vi "ReportEnd_A131258.vi"(6 "文件重命名":bool, 8 "error in (no error)":errorcluster caption="错误输入（无错误）", 10 "文件名称":string, 11 "report in":refnum<class "NI_report.lvclass"> caption="报表输入") -> (0 "error out":errorcluster caption="错误输出")   [LabVIEW 2020]
uses:
  <vilib>/Utility/NIReport.llb/NI_report.lvclass
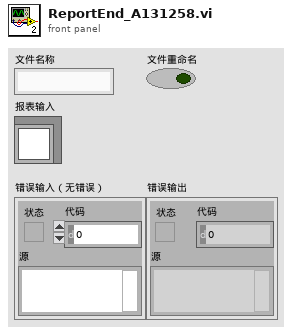
[diagram p1: front panel]
types:
  T1 = cluster{"Italic":enum16{"Italic Unchanged", "Italic On", "Italic Off"}, "Strike Through":enum16{"Strike Through Unchanged", "Strike Through On", "Strike Through Off"}, "Underline":enum16{"Underline Unchanged", "Underline On", "Underline Off"}, "Bold":enum16{"Bold Unchanged", "Bold On", "Bold Off"}}
  T2 = cluster{"Charset (-1)":i16, "Weight (-1)":i16, "Name":string, "Size":string}
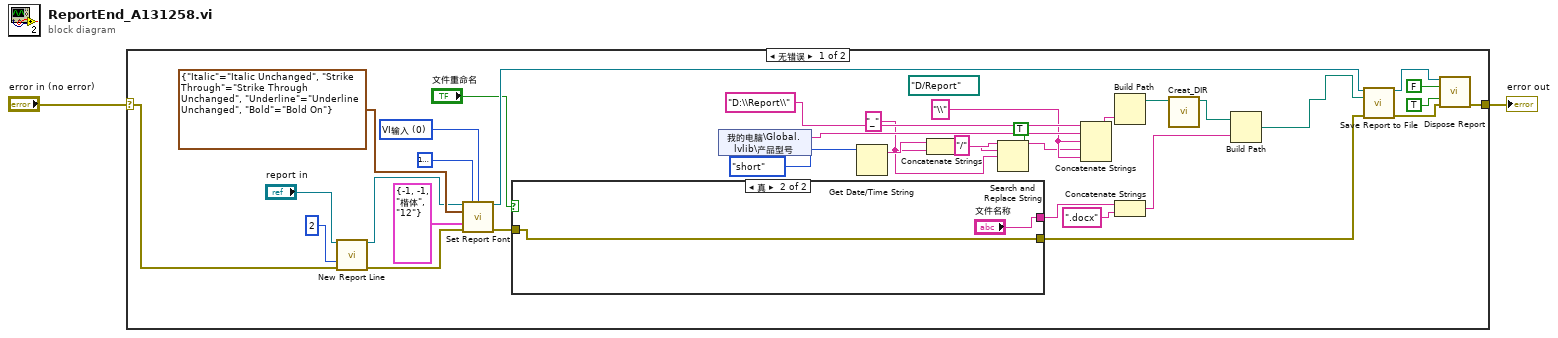
[diagram p0: block diagram]
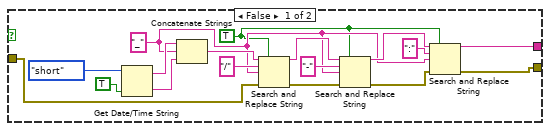
[diagram p2: hidden frame]
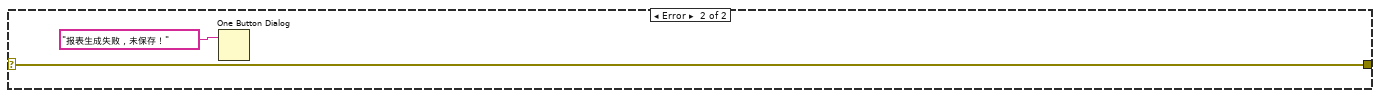
[diagram p3: hidden frame]
diagram:
  n1 = case shown="无错误" "error in (no error)" {
    selector: "error in (no error)" -> [w22 w58]
    tunnel: [w21 w58] -> w1
    frame No Error {
      w4 = "\\" ("替换字符串(\"\")")
      w7 = "_" ("替换字符串(\"\")")
      (unwired) path "D:/Report" ("report file path")
      w32 = u16 0 items=["VI输入", "字体对话框"] ("font settings source")
      n2 = call-dynamic "New Report Line.vi"("report in"="report in", "number of lines (1)"=2, "error in (no error)"=w22) -> ("report out"=w29:refnum<class "NI_report.lvclass">, "error out"=w28:errorcluster)  [unwired: 11 in]
      n3 = call-dynamic "Set Report Font.vi"("report in"=w29, "text color (unchanged)"=u32 16777224, "font settings source (VI Inputs)"=w32, "text options"=T1 {"Italic"=enum."Italic Unchanged", "Strike Through"=enum."Strike Through Unchanged", "Underline"=enum."Underline Unchanged", "Bold"=enum."Bold On"}, "font settings"=T2 {"Charset (-1)"=-1, "Weight (-1)"=-1, "Name"="楷体", "Size"="12"}, "error in (no error)"=w28) -> ("report out"=w25:refnum<class "NI_report.lvclass">, "error out"=w24:errorcluster)  [unwired: 7 in, 1 out]
      n4 = case shown="真" "文件重命名" {
        tunnel: [w49 "文件名称"] -> w19
        tunnel: w24 -> [w41 w55]
        tunnel: [w38 w55] -> w23
        frame False {
          w43 = TRUE ("替换全部？(F)")
          w44 = "_" ("替换字符串(\"\")")
          n5 = Get Date/Time String(date format (0)=enum16{"short", "long", "abbreviated"}."short" ("日期格式(0)"), want seconds? (F)=TRUE ("需要秒？(F)")) -> (date string=w54:string, time string=w50:string)  [unwired: 1 in]
          n6 = Concatenate Strings(w54, w44, w50) -> (w47:string)
          n7 = Search and Replace String(replace all?=w43, input string=w47, search string="/" ("搜索字符串"), replace string=w44, error in=w41) -> (result string=w46:string, error out=w40:errorcluster)  [unwired: 3 in, 2 out]
          n8 = Search and Replace String(replace all?=w43, input string=w46, search string="-" ("搜索字符串"), replace string=w44, error in=w40) -> (result string=w52:string, error out=w39:errorcluster)  [unwired: 3 in, 2 out]
          n9 = Search and Replace String(replace all?=w43, input string=w52, search string=":" ("搜索字符串"), replace string=w44, error in=w39) -> (result string=w49:string, error out=w38:errorcluster)  [unwired: 3 in, 2 out]
        }
        frame True {
        }
      }
      n10 = shared-variable "我的电脑\\Global.lvlib\\产品型号"() -> (w12:string)  [unwired: 1 in, 1 out]
      n11 = Get Date/Time String(date format (0)=enum16{"short", "long", "abbreviated"}."short" ("日期格式(0)")) -> (date string=w11:string)  [unwired: 2 in, 1 out]
      n12 = Concatenate Strings(w11, w7) -> (w10:string)
      n13 = Search and Replace String(replace all?=TRUE ("替换全部？(F)"), input string=w10, search string="/" ("搜索字符串"), replace string=w7) -> (result string=w3:string)  [unwired: 4 in, 3 out]
      n14 = Concatenate Strings("D:\\Report\\", w12, w4, w3, w4) -> (w5:string)
      n15 = Build Path(name or relative path=w5) -> (appended path=w17:path)  [unwired: 1 in]
      n16 = Concatenate Strings(w19, ".docx" ("字符串")) -> (w15:string)
      n17 = call "Creat_DIR.vi"("path"=w17) -> ("created path"=w16:path)  [unwired: 10 in]
      n18 = Build Path(base path=w16, name or relative path=w15) -> (appended path=w14:path)
      n19 = call-dynamic "Save Report to File.vi"("report in"=w25, "report file path"=w14, "error in (no error)"=w23) -> ("report out"=w37:refnum<class "NI_report.lvclass">, "error out"=w36:errorcluster)  [unwired: 11 in]
      n20 = call-dynamic "Dispose Report.vi"("report in"=w37, "wait until printing completed? (T)"=FALSE, "save changes? (F)"=TRUE, "error in (no error)"=w36) -> ("error out"=w21:errorcluster)  [unwired: 11 in]
    }
    frame Error {
      n21 = One Button Dialog(message="报表生成失败，未保存！" ("消息")) -> ()  [unwired: 1 in, 1 out]
    }
  }
  "error out" <- w1
